vi "output.vi"(8 "error in":errorcluster, 10 "data table in":T1, 11 "Scan Engine runtime in":refnum<class "Scan Engine runtime.lvclass">) -> (0 "error out":errorcluster, 2 "data table out":T1, 3 "Scan Engine runtime out":refnum<class "Scan Engine runtime.lvclass">)   [LabVIEW 2015, in "Scan Engine runtime.lvclass"]
doc: "Provides an interface for writing data to a module at runtime. While this interface performs no operations, a child should provide an override which may write to any open sessions, references, or interfaces."
uses:
  Scan Engine runtime.lvclass
  <vilib>/NI/Tag Bus/table/data table.ctl
  Scan Engine runtime.lvclass/Scan Engine runtime.ctl
  <vilib>/NI/Tag Bus/table/data polymorphs/read one/read Double.vi
  <vilib>/NI/Tag Bus/table/data polymorphs/read one/read Single.vi
  <vilib>/NI/Tag Bus/table/data polymorphs/read one/read I64.vi
  <vilib>/NI/Tag Bus/table/data polymorphs/read one/read I32.vi
  <vilib>/NI/Tag Bus/table/data polymorphs/read one/read I16.vi
  <vilib>/NI/Tag Bus/table/data polymorphs/read one/read I8.vi
  <vilib>/NI/Tag Bus/table/data polymorphs/read one/read U64.vi
  <vilib>/NI/Tag Bus/table/data polymorphs/read one/read U32.vi
  <vilib>/NI/Tag Bus/table/data polymorphs/read one/read U16.vi
  <vilib>/NI/Tag Bus/table/data polymorphs/read one/read U8.vi
  <vilib>/NI/Tag Bus/table/data polymorphs/read one/read Boolean.vi
  <vilib>/NI/Tag Bus/table/data polymorphs/read many/read Doubles.vi
  <vilib>/NI/Tag Bus/table/data polymorphs/read many/read Singles.vi
  <vilib>/NI/Tag Bus/table/data polymorphs/read many/read I64s.vi
  <vilib>/NI/Tag Bus/table/data polymorphs/read many/read I32s.vi
  <vilib>/NI/Tag Bus/table/data polymorphs/read many/read I16s.vi
  <vilib>/NI/Tag Bus/table/data polymorphs/read many/read I8s.vi
  <vilib>/NI/Tag Bus/table/data polymorphs/read many/read U64s.vi
  <vilib>/NI/Tag Bus/table/data polymorphs/read many/read U32s.vi
  <vilib>/NI/Tag Bus/table/data polymorphs/read many/read U16s.vi
  <vilib>/NI/Tag Bus/table/data polymorphs/read many/read U8s.vi
  <vilib>/NI/Tag Bus/table/data polymorphs/read many/read Booleans.vi
  <vilib>/NI/Tag Bus/table/data table.lvlib
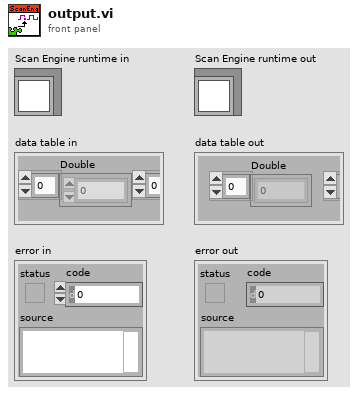
[diagram p1: front panel]
types:
  T1 = typedef "tag bus.lvlib/data table.lvlib/data table.ctl" = cluster{"Double":dbl[], "Single":sgl[], "I64":i64[], "I32":i32[], "I16":i16[], "I8":i8[], "U64":u64[], "U32":u32[], "U16":u16[], "U8":u8[], "Boolean":bool[], "String":string[], "Array of Double":cluster{"DBL Array":dbl[]}[], "Array of Single":cluster{"SGL Array":sgl[]}[], "Array of I64":cluster{"I64 Array":i64[]}[], "Array of I32":cluster{"I32 Array":i32[]}[], "Array of I16":cluster{"I16 Array":i16[]}[], "Array of I8":cluster{"I8 Array":i8[]}[], "Array of U64":cluster{"U64 Array":u64[]}[], "Array of U32":cluster{"U32 Array":u32[]}[], "Array of U16":cluster{"U16 Array":u16[]}[], "Array of U8":cluster{"U8 Array":u8[]}[], "Array of Boolean":cluster{"Boolean Array":bool[]}[], "Array of String":cluster{"String Array":string[]}[]}
  T2 = typedef "IO_index_map.ctl" = cluster{"module_ref":refnum<k21>, "data type":T3, "IO_variable_info":T4[], "IO_module_index_array":i32[], "IO_table_index":i32[], "IO_table_index_ordered":i32[], "use_scanned_methods":bool}
  T3 = typedef "tag bus.lvlib/tag descriptor.lvclass/Data Type.ctl" = enum16{"Double", "Single", "I64", "I32", "I16", "I8", "U64", "U32", "U16", "U8", "Boolean", "String", "Array of Double", "Array of Single", "Array of I64", "Array of I32", "Array of I16", "Array of I8", "Array of U64", "Array of U32", "Array of U16", "Array of U8", "Array of Boolean", "Array of String"}
  T4 = typedef "Scan Engine runtime.lvclass/Index Map.ctl" = cluster{"data type":T3, "variable ref":refnum<k21>, "index":i32, "IO Var":bool, "module_index":i32}
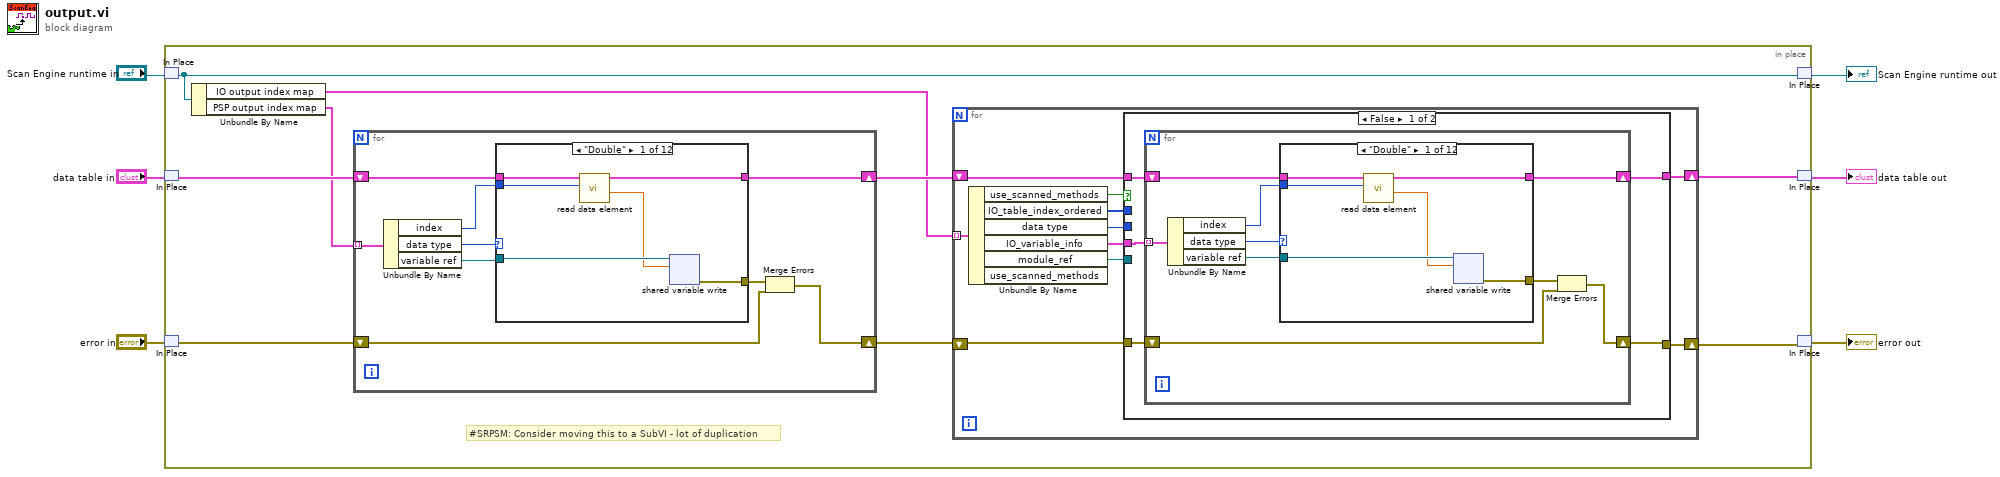
[diagram p0: block diagram]
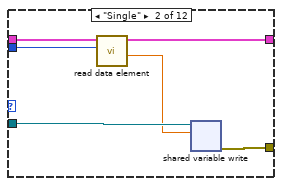
[diagram p2: hidden frame]
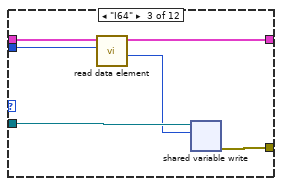
[diagram p3: hidden frame]
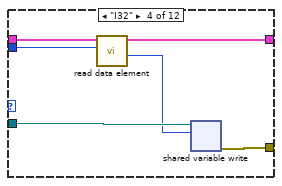
[diagram p4: hidden frame]
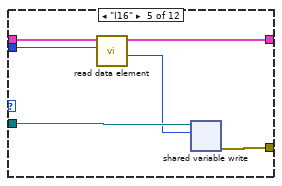
[diagram p5: hidden frame]
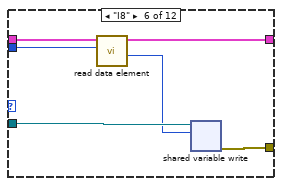
[diagram p6: hidden frame]
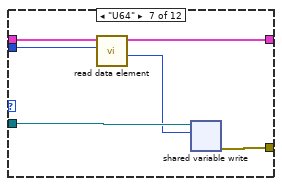
[diagram p7: hidden frame]
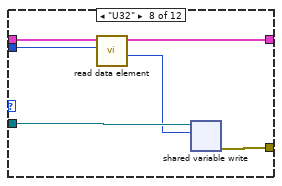
[diagram p8: hidden frame]
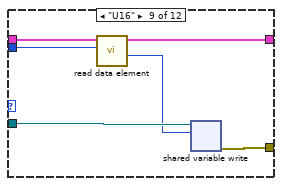
[diagram p9: hidden frame]
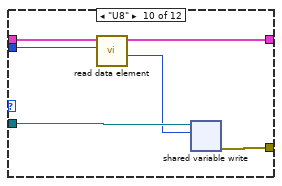
[diagram p10: hidden frame]
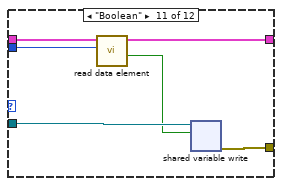
[diagram p11: hidden frame]
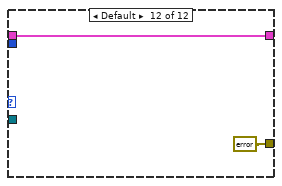
[diagram p12: hidden frame]
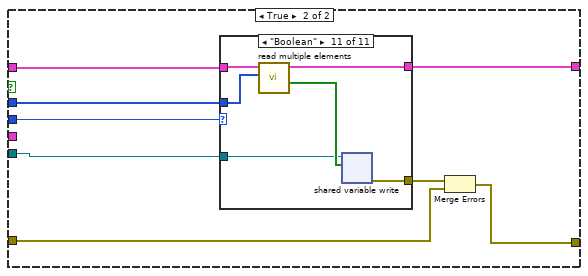
[diagram p13: hidden frame]
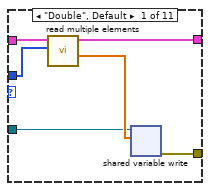
[diagram p14: hidden frame]
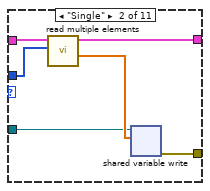
[diagram p15: hidden frame]
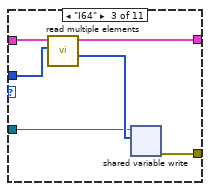
[diagram p16: hidden frame]
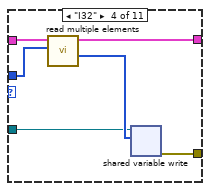
[diagram p17: hidden frame]
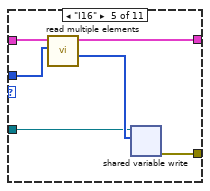
[diagram p18: hidden frame]
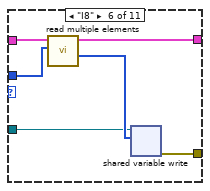
[diagram p19: hidden frame]
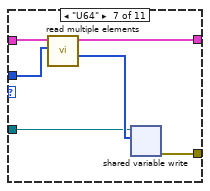
[diagram p20: hidden frame]
diagram:
  n1 = in-place {
    # "#SRPSM: Consider moving this to a SubVI - lot of duplication"
    n2 = in-place-match #1("Scan Engine runtime in") -> (w15:refnum<class "Scan Engine runtime.lvclass">)
    n3 = in-place-match #2("data table in") -> (w14:T1)
    n4 = in-place-match #3("error in") -> (w12:errorcluster)
    n5 = Unbundle By Name(w15) -> ("IO output index map"=w9:T2[], "PSP output index map"=w13:T4[])
    n6 = for {
      shift-right: [w187] -> w11
      shift-left: w14 -> [w188]
      tunnel: w13 -> [w190] mode=indexing
      shift-right: [w182] -> w10
      shift-left: w12 -> [w183]
      n7 = Unbundle By Name(w190) -> ("index"=w185:i32, "data type"=w189:T3, "variable ref"=w186:refnum<k21>)
      n8 = case shown="\"Double\"" w189 {
        tunnel: w188 -> [w195 w201 w207 w213 w219 w225 w231 w237 w243 w249 w255 w258]
        tunnel: [w193 w199 w205 w211 w217 w223 w229 w235 w241 w247 w253 w258] -> w187
        tunnel: w186 -> [w192 w198 w204 w210 w216 w222 w228 w234 w240 w246 w252 _]
        tunnel: [w196 w202 w208 w214 w220 w226 w232 w238 w244 w250 w256 errorcluster {"status"=FALSE, "code"=0, "source"=""} ("error IO")] -> w184
        tunnel: w185 -> [w194 w200 w206 w212 w218 w224 w230 w236 w242 w248 w254 _]
        frame "Double" {
          n9 = call-poly <vilib>:"read data element.vi"("index"=w194, "data table in"=w195) -> ("value"=w191:dbl, "data table out"=w193:T1)  [unwired: 8 in]
          n10 = shared-variable-write(w192, w191) -> (w196:errorcluster)  [unwired: 1 in, 1 out]
        }
        frame "Single" {
          n11 = call-poly <vilib>:"read data element.vi"("index"=w200, "data table in"=w201) -> ("value"=w197:sgl, "data table out"=w199:T1)  [unwired: 8 in]
          n12 = shared-variable-write(w198, w197) -> (w202:errorcluster)  [unwired: 1 in, 1 out]
        }
        frame "I64" {
          n13 = call-poly <vilib>:"read data element.vi"("index"=w206, "data table in"=w207) -> ("value"=w203:i64, "data table out"=w205:T1)  [unwired: 8 in]
          n14 = shared-variable-write(w204, w203) -> (w208:errorcluster)  [unwired: 1 in, 1 out]
        }
        frame "I32" {
          n15 = call-poly <vilib>:"read data element.vi"("index"=w212, "data table in"=w213) -> ("value"=w209:i32, "data table out"=w211:T1)  [unwired: 8 in]
          n16 = shared-variable-write(w210, w209) -> (w214:errorcluster)  [unwired: 1 in, 1 out]
        }
        frame "I16" {
          n17 = call-poly <vilib>:"read data element.vi"("index"=w218, "data table in"=w219) -> ("value"=w215:i16, "data table out"=w217:T1)  [unwired: 8 in]
          n18 = shared-variable-write(w216, w215) -> (w220:errorcluster)  [unwired: 1 in, 1 out]
        }
        frame "I8" {
          n19 = call-poly <vilib>:"read data element.vi"("index"=w224, "data table in"=w225) -> ("value"=w221:i8, "data table out"=w223:T1)  [unwired: 8 in]
          n20 = shared-variable-write(w222, w221) -> (w226:errorcluster)  [unwired: 1 in, 1 out]
        }
        frame "U64" {
          n21 = call-poly <vilib>:"read data element.vi"("index"=w230, "data table in"=w231) -> ("value"=w227:u64, "data table out"=w229:T1)  [unwired: 8 in]
          n22 = shared-variable-write(w228, w227) -> (w232:errorcluster)  [unwired: 1 in, 1 out]
        }
        frame "U32" {
          n23 = call-poly <vilib>:"read data element.vi"("index"=w236, "data table in"=w237) -> ("value"=w233:u32, "data table out"=w235:T1)  [unwired: 8 in]
          n24 = shared-variable-write(w234, w233) -> (w238:errorcluster)  [unwired: 1 in, 1 out]
        }
        frame "U16" {
          n25 = call-poly <vilib>:"read data element.vi"("index"=w242, "data table in"=w243) -> ("value"=w239:u16, "data table out"=w241:T1)  [unwired: 8 in]
          n26 = shared-variable-write(w240, w239) -> (w244:errorcluster)  [unwired: 1 in, 1 out]
        }
        frame "U8" {
          n27 = call-poly <vilib>:"read data element.vi"("index"=w248, "data table in"=w249) -> ("value"=w245:u8, "data table out"=w247:T1)  [unwired: 8 in]
          n28 = shared-variable-write(w246, w245) -> (w250:errorcluster)  [unwired: 1 in, 1 out]
        }
        frame "Boolean" {
          n29 = call-poly <vilib>:"read data element.vi"("index"=w254, "data table in"=w255) -> ("value"=w251:bool, "data table out"=w253:T1)  [unwired: 8 in]
          n30 = shared-variable-write(w252, w251) -> (w256:errorcluster)  [unwired: 1 in, 1 out]
        }
        frame Default {
        }
      }
      n31 = Merge Errors(w184, w183) -> (w182:errorcluster)
    }
    n32 = for {
      tunnel: w9 -> [w25] mode=indexing
      shift-right: [w19] -> w8
      shift-left: w10 -> [w20]
      shift-right: [w16] -> w7
      shift-left: w11 -> [w24]
      n33 = Unbundle By Name(w25) -> ("use_scanned_methods"=w22:bool, "IO_table_index_ordered"=w23:i32[], "data type"=w17:T3, "IO_variable_info"=w21:T4[], "module_ref"=w18:refnum<k21>)  [unwired: 1 out]
      n34 = case shown="False" w22 {
        tunnel: w24 -> [w30 w115]
        tunnel: w23 -> [_ w109]
        tunnel: w21 -> [w29 _]
        tunnel: w20 -> [w28 w113]
        tunnel: [w27 w112] -> w19
        tunnel: w18 -> [_ w111]
        tunnel: w17 -> [_ w110]
        tunnel: [w26 w108] -> w16
        frame False {
          n35 = for {
            shift-right: [w36] -> w26
            shift-left: w30 -> [w37]
            tunnel: w29 -> [w39] mode=indexing
            shift-right: [w31] -> w27
            shift-left: w28 -> [w32]
            n36 = Unbundle By Name(w39) -> ("index"=w34:i32, "data type"=w38:T3, "variable ref"=w35:refnum<k21>)
            n37 = case shown="\"Double\"" w38 {
              tunnel: w37 -> [w44 w50 w56 w62 w68 w74 w80 w86 w92 w98 w104 w107]
              tunnel: [w42 w48 w54 w60 w66 w72 w78 w84 w90 w96 w102 w107] -> w36
              tunnel: w35 -> [w41 w47 w53 w59 w65 w71 w77 w83 w89 w95 w101 _]
              tunnel: [w45 w51 w57 w63 w69 w75 w81 w87 w93 w99 w105 errorcluster {"status"=FALSE, "code"=0, "source"=""} ("error IO")] -> w33
              tunnel: w34 -> [w43 w49 w55 w61 w67 w73 w79 w85 w91 w97 w103 _]
              frame "Double" {
                n38 = call-poly <vilib>:"read data element.vi"("index"=w43, "data table in"=w44) -> ("value"=w40:dbl, "data table out"=w42:T1)  [unwired: 8 in]
                n39 = shared-variable-write(w41, w40) -> (w45:errorcluster)  [unwired: 1 in, 1 out]
              }
              frame "Single" {
                n40 = call-poly <vilib>:"read data element.vi"("index"=w49, "data table in"=w50) -> ("value"=w46:sgl, "data table out"=w48:T1)  [unwired: 8 in]
                n41 = shared-variable-write(w47, w46) -> (w51:errorcluster)  [unwired: 1 in, 1 out]
              }
              frame "I64" {
                n42 = call-poly <vilib>:"read data element.vi"("index"=w55, "data table in"=w56) -> ("value"=w52:i64, "data table out"=w54:T1)  [unwired: 8 in]
                n43 = shared-variable-write(w53, w52) -> (w57:errorcluster)  [unwired: 1 in, 1 out]
              }
              frame "I32" {
                n44 = call-poly <vilib>:"read data element.vi"("index"=w61, "data table in"=w62) -> ("value"=w58:i32, "data table out"=w60:T1)  [unwired: 8 in]
                n45 = shared-variable-write(w59, w58) -> (w63:errorcluster)  [unwired: 1 in, 1 out]
              }
              frame "I16" {
                n46 = call-poly <vilib>:"read data element.vi"("index"=w67, "data table in"=w68) -> ("value"=w64:i16, "data table out"=w66:T1)  [unwired: 8 in]
                n47 = shared-variable-write(w65, w64) -> (w69:errorcluster)  [unwired: 1 in, 1 out]
              }
              frame "I8" {
                n48 = call-poly <vilib>:"read data element.vi"("index"=w73, "data table in"=w74) -> ("value"=w70:i8, "data table out"=w72:T1)  [unwired: 8 in]
                n49 = shared-variable-write(w71, w70) -> (w75:errorcluster)  [unwired: 1 in, 1 out]
              }
              frame "U64" {
                n50 = call-poly <vilib>:"read data element.vi"("index"=w79, "data table in"=w80) -> ("value"=w76:u64, "data table out"=w78:T1)  [unwired: 8 in]
                n51 = shared-variable-write(w77, w76) -> (w81:errorcluster)  [unwired: 1 in, 1 out]
              }
              frame "U32" {
                n52 = call-poly <vilib>:"read data element.vi"("index"=w85, "data table in"=w86) -> ("value"=w82:u32, "data table out"=w84:T1)  [unwired: 8 in]
                n53 = shared-variable-write(w83, w82) -> (w87:errorcluster)  [unwired: 1 in, 1 out]
              }
              frame "U16" {
                n54 = call-poly <vilib>:"read data element.vi"("index"=w91, "data table in"=w92) -> ("value"=w88:u16, "data table out"=w90:T1)  [unwired: 8 in]
                n55 = shared-variable-write(w89, w88) -> (w93:errorcluster)  [unwired: 1 in, 1 out]
              }
              frame "U8" {
                n56 = call-poly <vilib>:"read data element.vi"("index"=w97, "data table in"=w98) -> ("value"=w94:u8, "data table out"=w96:T1)  [unwired: 8 in]
                n57 = shared-variable-write(w95, w94) -> (w99:errorcluster)  [unwired: 1 in, 1 out]
              }
              frame "Boolean" {
                n58 = call-poly <vilib>:"read data element.vi"("index"=w103, "data table in"=w104) -> ("value"=w100:bool, "data table out"=w102:T1)  [unwired: 8 in]
                n59 = shared-variable-write(w101, w100) -> (w105:errorcluster)  [unwired: 1 in, 1 out]
              }
              frame Default {
              }
            }
            n60 = Merge Errors(w33, w32) -> (w31:errorcluster)
          }
        }
        frame True {
          n61 = case shown="\"Boolean\"" w110 {
            tunnel: w115 -> [w121 w127 w133 w139 w145 w151 w157 w163 w169 w175 w181]
            tunnel: w111 -> [w119 w125 w131 w137 w143 w149 w155 w161 w167 w173 w179]
            tunnel: [w118 w124 w130 w136 w142 w148 w154 w160 w166 w172 w178] -> w114
            tunnel: w109 -> [w117 w123 w129 w135 w141 w147 w153 w159 w165 w171 w177]
            tunnel: [w116 w122 w128 w134 w140 w146 w152 w158 w164 w170 w176] -> w108
            frame "Double", Default {
              n62 = call-poly <vilib>:"read multiple elements.vi"("indices"=w117, "data table in"=w121) -> ("values"=w120:dbl[], "data table out"=w116:T1)  [unwired: 8 in]
              n63 = shared-variable-write(w119, w120) -> (w118:errorcluster)  [unwired: 1 in, 1 out]
            }
            frame "Single" {
              n64 = call-poly <vilib>:"read multiple elements.vi"("indices"=w123, "data table in"=w127) -> ("values"=w126:sgl[], "data table out"=w122:T1)  [unwired: 8 in]
              n65 = shared-variable-write(w125, w126) -> (w124:errorcluster)  [unwired: 1 in, 1 out]
            }
            frame "I64" {
              n66 = call-poly <vilib>:"read multiple elements.vi"("indices"=w129, "data table in"=w133) -> ("values"=w132:i64[], "data table out"=w128:T1)  [unwired: 8 in]
              n67 = shared-variable-write(w131, w132) -> (w130:errorcluster)  [unwired: 1 in, 1 out]
            }
            frame "I32" {
              n68 = call-poly <vilib>:"read multiple elements.vi"("indices"=w135, "data table in"=w139) -> ("values"=w138:i32[], "data table out"=w134:T1)  [unwired: 8 in]
              n69 = shared-variable-write(w137, w138) -> (w136:errorcluster)  [unwired: 1 in, 1 out]
            }
            frame "I16" {
              n70 = call-poly <vilib>:"read multiple elements.vi"("indices"=w141, "data table in"=w145) -> ("values"=w144:i16[], "data table out"=w140:T1)  [unwired: 8 in]
              n71 = shared-variable-write(w143, w144) -> (w142:errorcluster)  [unwired: 1 in, 1 out]
            }
            frame "I8" {
              n72 = call-poly <vilib>:"read multiple elements.vi"("indices"=w147, "data table in"=w151) -> ("values"=w150:i8[], "data table out"=w146:T1)  [unwired: 8 in]
              n73 = shared-variable-write(w149, w150) -> (w148:errorcluster)  [unwired: 1 in, 1 out]
            }
            frame "U64" {
              n74 = call-poly <vilib>:"read multiple elements.vi"("indices"=w153, "data table in"=w157) -> ("values"=w156:u64[], "data table out"=w152:T1)  [unwired: 8 in]
              n75 = shared-variable-write(w155, w156) -> (w154:errorcluster)  [unwired: 1 in, 1 out]
            }
            frame "U32" {
              n76 = call-poly <vilib>:"read multiple elements.vi"("indices"=w159, "data table in"=w163) -> ("values"=w162:u32[], "data table out"=w158:T1)  [unwired: 8 in]
              n77 = shared-variable-write(w161, w162) -> (w160:errorcluster)  [unwired: 1 in, 1 out]
            }
            frame "U16" {
              n78 = call-poly <vilib>:"read multiple elements.vi"("indices"=w165, "data table in"=w169) -> ("values"=w168:u16[], "data table out"=w164:T1)  [unwired: 8 in]
              n79 = shared-variable-write(w167, w168) -> (w166:errorcluster)  [unwired: 1 in, 1 out]
            }
            frame "U8" {
              n80 = call-poly <vilib>:"read multiple elements.vi"("indices"=w171, "data table in"=w175) -> ("values"=w174:u8[], "data table out"=w170:T1)  [unwired: 8 in]
              n81 = shared-variable-write(w173, w174) -> (w172:errorcluster)  [unwired: 1 in, 1 out]
            }
            frame "Boolean" {
              n82 = call-poly <vilib>:"read multiple elements.vi"("indices"=w177, "data table in"=w181) -> ("values"=w180:bool[], "data table out"=w176:T1)  [unwired: 8 in]
              n83 = shared-variable-write(w179, w180) -> (w178:errorcluster)  [unwired: 1 in, 1 out]
            }
          }
          n84 = Merge Errors(w114, w113) -> (w112:errorcluster)
        }
      }
    }
    n85 = in-place-match #1(w15) -> (→"Scan Engine runtime out":refnum<class "Scan Engine runtime.lvclass">)
    n86 = in-place-match #2(w7) -> (→"data table out":T1)
    n87 = in-place-match #3(w8) -> (→"error out":errorcluster)
  }
